vi "SetChannel.vi"(4 "error in":errorcluster, 5 "Channel 1 or 2":string, 6 "Device Key In":string, 7 "PM Cmds In":refnum<k24>) -> (0 "error out":errorcluster, 2 "Device Key Out":string, 3 "PM Cmds Out":refnum<k24>)   [LabVIEW 2021]
uses:
  C:/_git/mantoles-dev-box/LabVIEW/sample-code/LabVIEW 2010/PowerMeterCommands.dll
  PowerMeterCommands.dll
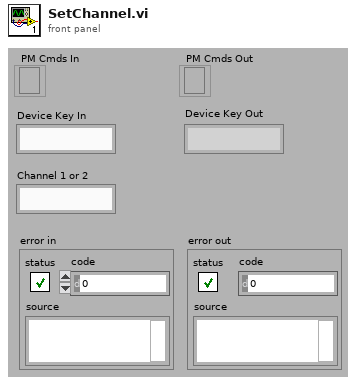
[diagram p1: front panel]
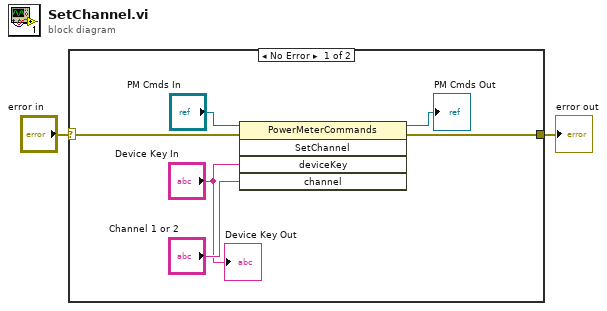
[diagram p0: block diagram]
diagram:
  n1 = case shown="No Error" "error in" {
    selector: "error in" -> [w4 w9]
    tunnel: [w6 w9] -> w2
    frame No Error {
      n2 = invoke class="PowerMeterCommands" method="SetChannel"(reference="PM Cmds In", error in=w4, "deviceKey"="Device Key In", "channel"="Channel 1 or 2") -> (reference out=→"PM Cmds Out":refnum<k24>, error out=w6:errorcluster)  [unwired: 1 in, 3 out]
      "Device Key Out" <- "Device Key In"
    }
    frame Error {
    }
  }
  "error out" <- w2
